vi "myRIO_BRig_RT_dataCurrent_count_generic__increment.vi"(10 "input_increment":i32, 11 "input_dataCurrent":u16[](array[numeric])) -> (0 "output_count_generic":i32, 1 "output_thresholdReached":bool, 3 "output_dataCurrent":u16[](array[numeric]))   [LabVIEW 2014]
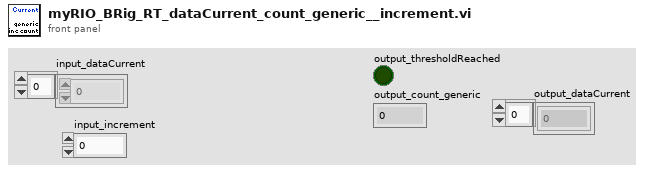
[diagram p1: front panel]
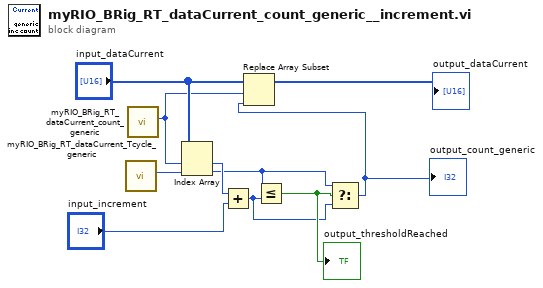
[diagram p0: block diagram]
diagram:
  n1 = call "myRIO_BRig_RT_dataCurrent_Tcycle_generic.vi"() -> ("output_Tcycle_generic"=w8:i32)  [unwired: 11 in]
  n2 = call "myRIO_BRig_RT_dataCurrent_count_generic.vi"() -> ("output_count_generic"=w9:i32)  [unwired: 11 in]
  n3 = Index Array(array="input_dataCurrent", index #1=w9, index #2=w8) -> (element #1=w6:u16, element #2=w3:u16)
  n4 = Add(x=w6, y="input_increment") -> (x+y=w4:i32)
  n5 = Less Or Equal?(x=w3, y=w4) -> (x <= y?=w5:bool)
  "output_thresholdReached" <- w5
  n6 = Select(t=w3, s=w5, f=w4) -> (s? t:f=w2:i32)
  "output_count_generic" <- w2
  n7 = Replace Array Subset(array="input_dataCurrent", new element=w2, index=w9) -> (→"output_dataCurrent":u16[])
